vi "worksheet set row pixels.vi"(7 "format":u32, 8 "error in (no error)":errorcluster, 9 "pixels":u32, 10 "row":u32, 11 "worksheet":u32) -> (0 "error out":errorcluster, 3 "function return":u32(ring))   [LabVIEW 2015, in "xlsxwriter.lvlib"]
doc: "lxw_error worksheet_set_row_pixels(lxw_worksheet worksheet, lxw_row_t row, uint32_t pixels, lxw_format format);"
uses:
  xlsxwriter.lvlib
  xlsxwriter.dll
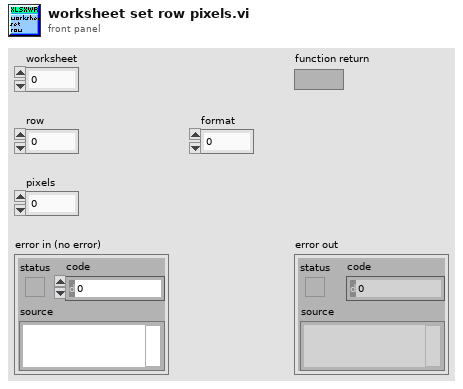
[diagram p1: front panel]
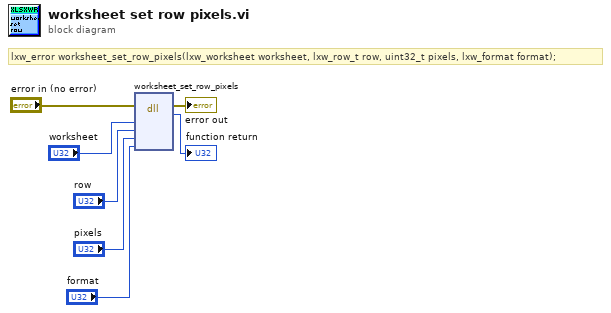
[diagram p0: block diagram]
diagram:
  # "lxw_error worksheet_set_row_pixels(lxw_worksheet worksheet, lxw_row_t row, uint32_t pixels, lxw_format format);"
  n1 = dll-call lib="C:/Users/WDAGUtilityAccount/Desktop/lv_vis_added_cell/xlsxwriter.*" fn="worksheet_set_row_pixels"(error in="error in (no error)", "worksheet"="worksheet", "row"="row", "pixels"="pixels", "format"="format") -> (error out=→"error out":errorcluster, →"function return":u32)  [unwired: 6 in, 1 out]
